vi "Atto DRY Interface is Controlling Temperature.vi"(8 "error in (no error)":errorcluster, 11 "ControllingTemperature":i32) -> (0 "error out":errorcluster, 2 "function return":i32, 3 "ControllingTemperature out":i32)   [LabVIEW 2016, in "attoDRYLib.lvlib"]
doc: "int32_t __cdecl AttoDRY_Interface_isControllingTemperature(\n int *ControllingTemperature);"
uses:
  <userlib>/attoDRYLib/attoDRYLib.lvlib
  <userlib>/attoDRYLib/attoDRYLib.dll
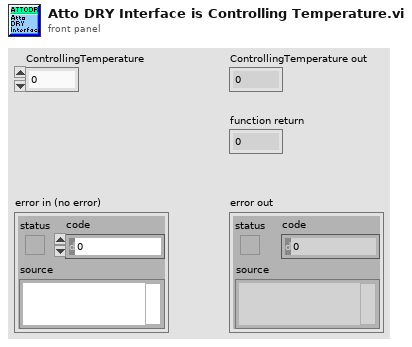
[diagram p1: front panel]
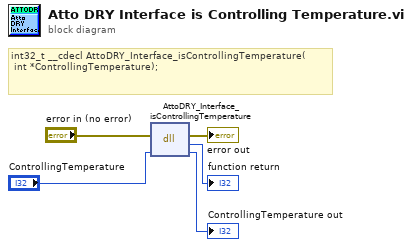
[diagram p0: block diagram]
diagram:
  # "int32_t __cdecl AttoDRY_Interface_isControllingTemperature(\n\tint *ControllingTemperature);"
  n1 = dll-call lib="C:/Program Files (x86)/National Instruments/LabVIEW 2016/user.lib/attoDRYLib/attoDRYLib.*" fn="AttoDRY_Interface_isControllingTemperature"(error in="error in (no error)", "ControllingTemperature"="ControllingTemperature") -> (error out=→"error out":errorcluster, →"function return":i32, "ControllingTemperature"=→"ControllingTemperature out":i32)  [unwired: 2 in, 1 out]
